vi "Ch_data_title_pattern (SubVI).vi"(8 "error in":errorcluster, 9 "Единица измерений":string) -> (0 "error out":errorcluster, 2 "Path":path, 3 "Byte Stream File out":refnum<file>)   [LabVIEW 2015]
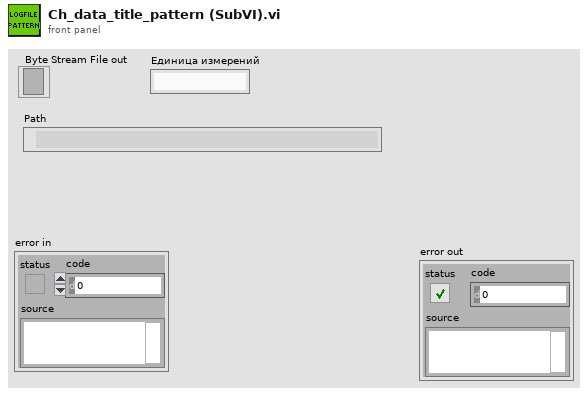
[diagram p1: front panel]
types:
  T1 = enum16{"open", "replace", "create", "open or create", "replace or create", "replace or create with confirmation"}
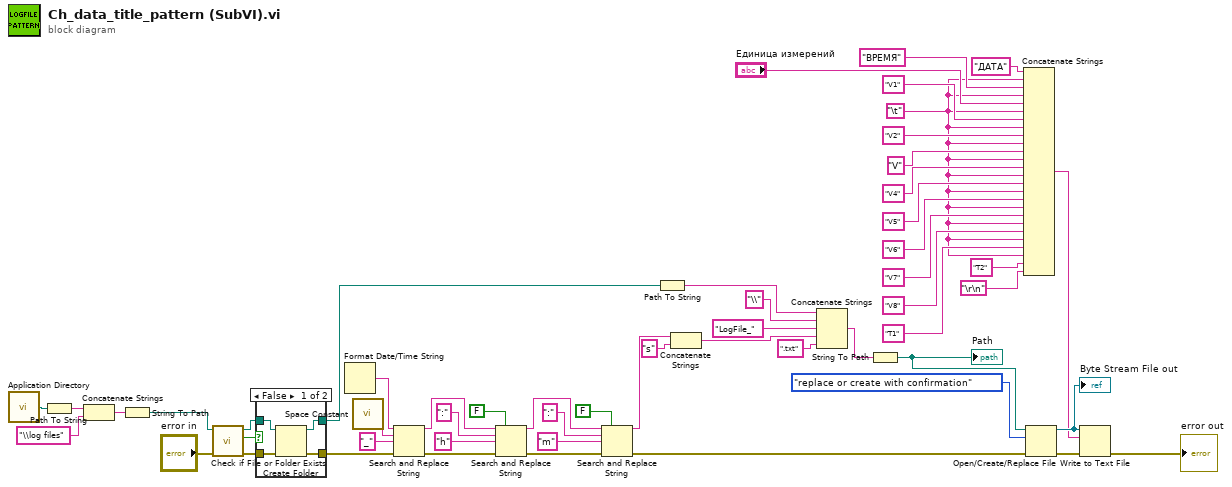
[diagram p0: block diagram]
diagram:
  w3 = "\t"
  n1 = call <vilib>:"Application Directory.vi"() -> ("Application Directory"=w13:path)
  n2 = Path To String(path=w13) -> (string=w12:string)
  n3 = Concatenate Strings(w12, "\\log files" ("replace string (\"\")")) -> (w10:string)
  n4 = String To Path(string=w10) -> (path=w9:path)
  n5 = call <vilib>:"Check if File or Folder Exists.vi"("error in (no error)"="error in", "path"=w9) -> ("error out"=w47:errorcluster, "file or folder exists?"=w46:bool, "dup path"=w48:path)  [unwired: 7 out]
  n6 = case shown="False" w46 {
    tunnel: [w58 w60] -> w14
    tunnel: w48 -> [w57 w60]
    tunnel: w47 -> [w56 w59]
    tunnel: [w55 w59] -> w15
    frame False {
      n7 = Create Folder(path (use dialog)=w57, error in=w56) -> (created path=w58:path, error out=w55:errorcluster)  [unwired: 2 out]
    }
    frame True {
    }
  }
  n8 = Format Date/Time String() -> (date/time string=w45:string)  [unwired: 3 out]
  n9 = call <vilib>:"Space Constant.vi"() -> ("String"=w26:string)
  n10 = Search and Replace String(input string=w45, search string=w26, replace string="_" ("replace string (\"\")"), error in=w15) -> (result string=w28:string, error out=w38:errorcluster)  [unwired: 6 out]
  n11 = Search and Replace String(replace all?=FALSE ("replace all? (F)"), input string=w28, search string=":", replace string="h" ("replace string (\"\")"), error in=w38) -> (result string=w35:string, error out=w39:errorcluster)  [unwired: 5 out]
  n12 = Search and Replace String(replace all?=FALSE ("replace all? (F)"), input string=w35, search string=":", replace string="m" ("replace string (\"\")"), error in=w39) -> (result string=w40:string, error out=w24:errorcluster)  [unwired: 5 out]
  n13 = Path To String(path=w14) -> (string=w36:string)
  n14 = Concatenate Strings(w40, "s" ("string")) -> (w43:string)
  n15 = Concatenate Strings(w36, "\\" ("string"), "LogFile_" ("string"), w43, ".txt" ("default name")) -> (w25:string)
  n16 = String To Path(string=w25) -> (path=w23:path)
  "Path" <- w23
  n17 = Concatenate Strings("ДАТА" ("string"), w3, "ВРЕМЯ" ("string"), w3, "Единица измерений", w3, "V1" ("string"), w3, "V2" ("string"), w3, "V" ("string"), w3, "V4" ("string"), w3, "V5" ("string"), w3, "V6" ("string"), w3, "V7" ("string"), w3, "V8" ("string"), w3, "T1" ("string"), w3, "T2" ("string"), "\r\n") -> (w50:string)
  n18 = Open/Create/Replace File(file path (use dialog)=w23, error in=w24, operation (0:open)=T1."replace or create with confirmation") -> (refnum out=w53:refnum<file>, error out=w51:errorcluster)  [unwired: 4 out]
  "Byte Stream File out" <- w53
  n19 = Write to Text File(file (use dialog)=w53, text=w50, error in=w51) -> (error out=→"error out":errorcluster)  [unwired: 3 out]
